vi "StringToArray_Sushu.vi"(10 "delimiter (Tab)":string, 11 "State Queue":string) -> (2 "Original array":string[](array[string]), 3 "Array":string[](array[string]), 5 "Final size(s)":i32, 7 "one row string":string)   [LabVIEW 2020, in "sushu.lvlib"]
doc: "字符串转换成数组。\n20131228\n蒋松：jiangsong@outlook.com\nsina：@sushu1051"
uses:
  <userlib>/sushu/sushu.lvlib
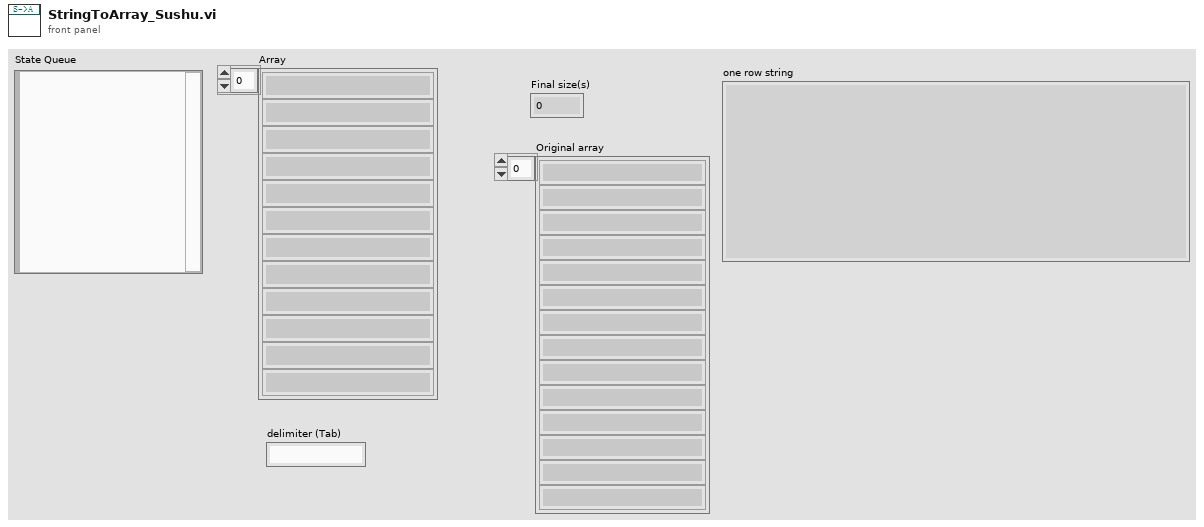
[diagram p1: front panel]
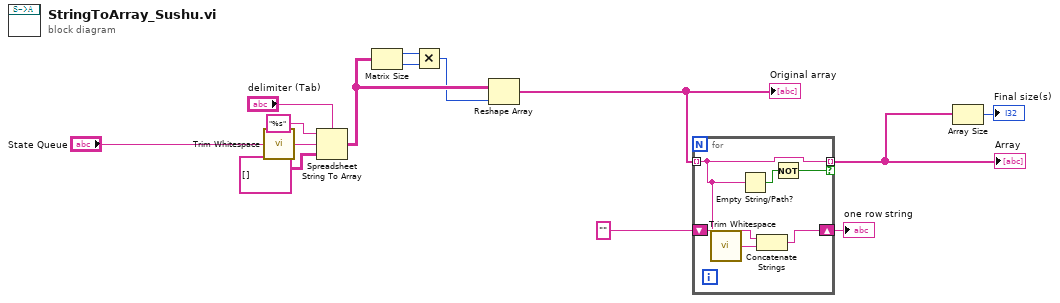
[diagram p0: block diagram]
diagram:
  n1 = call <vilib>:"Trim Whitespace.vi"("string"="State Queue") -> ("trimmed string"=w13:string)  [unwired: 1 in]
  n2 = Spreadsheet String To Array(delimiter (Tab)="delimiter (Tab)", format string="%s", spreadsheet string=w13, array type (2D Dbl)=string[][] []) -> (array=w4:string[][])
  n3 = Matrix Size(0:w4) -> (1:w5:i32, 2:w6:i32)
  n4 = Multiply(x=w5, y=w6) -> (x*y=w3:i32)
  n5 = Reshape Array(w4, w3) -> (w1:string[])
  "Original array" <- w1
  n6 = for {
    tunnel: w1 -> [w15] mode=indexing
    tunnel: [w15] -> w10 mode=indexing if=w19
    shift-right: [w17] -> w7
    shift-left: "" ("format string") -> [w18]
    n7 = call <vilib>:"Trim Whitespace.vi"("string"=w15) -> ("trimmed string"=w16:string)  [unwired: 1 in]
    n8 = Empty String/Path?(string/path=w15) -> (empty?=w20:bool)
    n9 = Concatenate Strings(w18, w16) -> (w17:string)
    n10 = Not(x=w20) -> (.not. x?=w19:bool)
  }
  "Array" <- w10
  "one row string" <- w7
  n11 = Array Size(array=w10) -> (size(s)=→"Final size(s)":i32)
